vi "Part 1.vi"(11 "Input":string) -> (3 "Output":i64)   [LabVIEW 2021]
panel:
  out "array":string[](array[string])
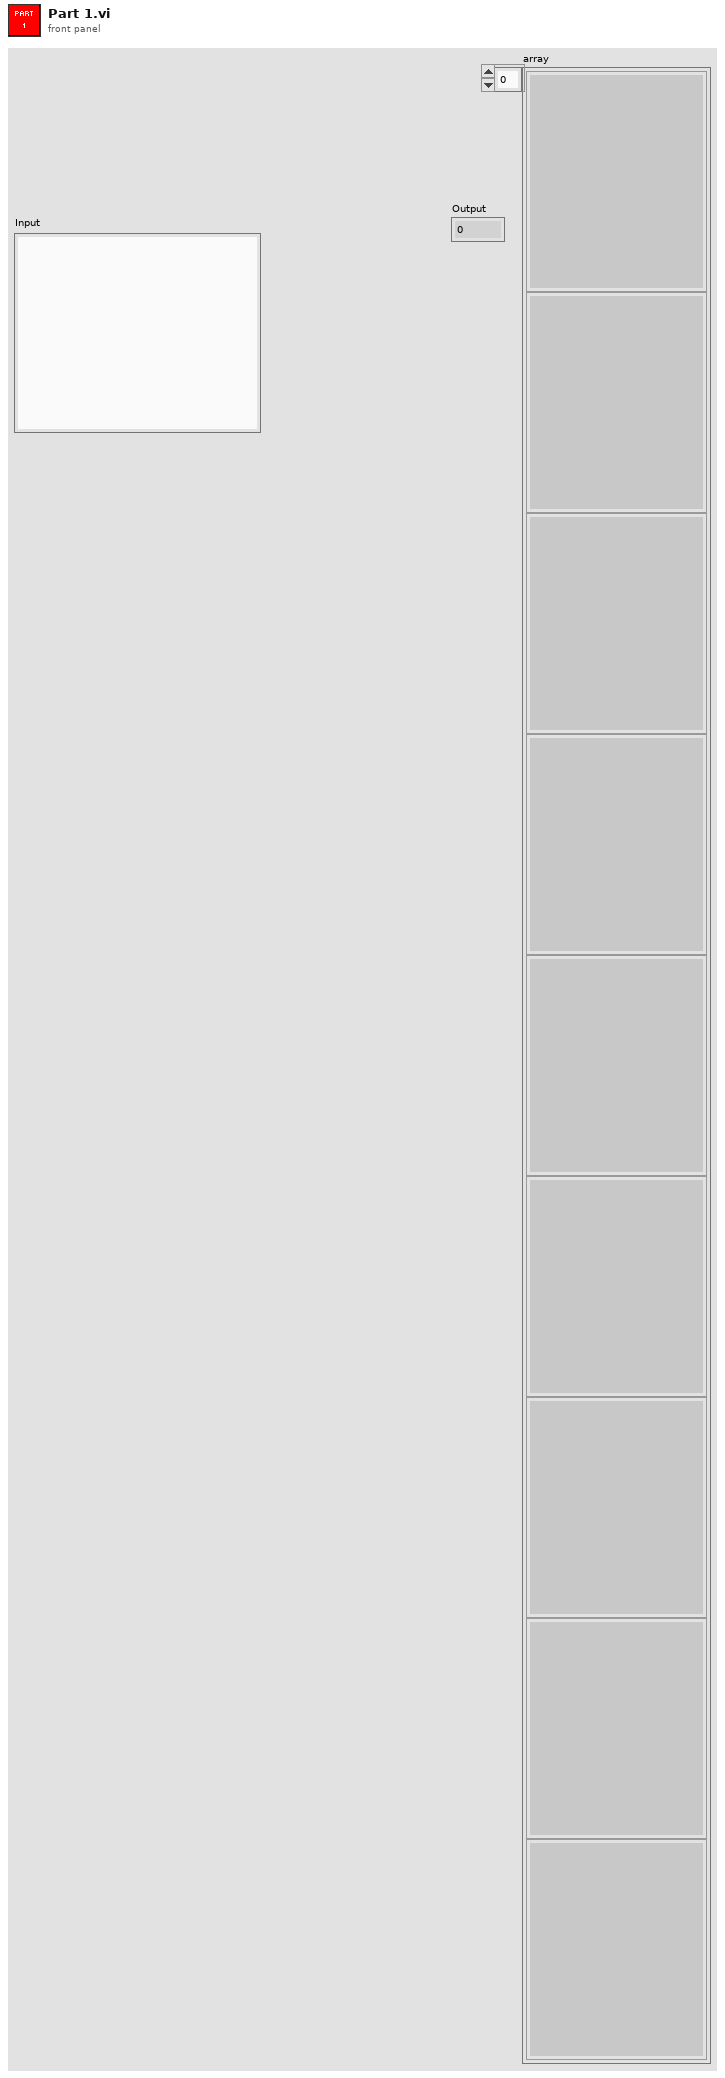
[diagram p1: front panel]
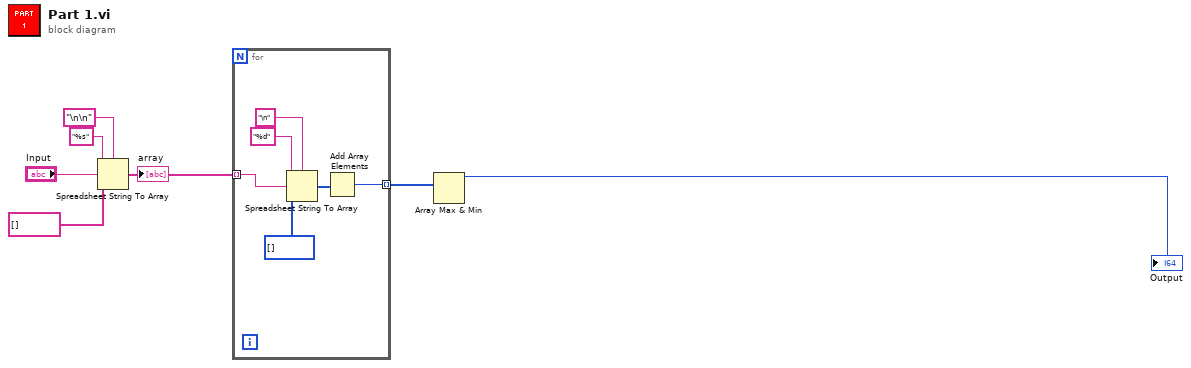
[diagram p0: block diagram]
diagram:
  n1 = Spreadsheet String To Array(delimiter (Tab)="\n\n", format string="%s", spreadsheet string="Input", array type (2D Dbl)=string[] []) -> (array=w3:string[])
  "array" <- w3
  n2 = for {
    tunnel: w3 -> [w11] mode=indexing
    tunnel: [w8] -> w2 mode=indexing
    n3 = Spreadsheet String To Array(delimiter (Tab)="\n", format string="%d", spreadsheet string=w11, array type (2D Dbl)=i64[] []) -> (array=w9:i64[])
    n4 = Add Array Elements(numeric array=w9) -> (sum=w8:i64)
  }
  n5 = Array Max & Min(array=w2) -> (max value=→"Output":i64)  [unwired: 3 out]
